vi "SubVI_Res_Result.vi"(8 "error in":errorcluster caption="에러 입력(에러 없음)", 11 "Q_data":T1) -> (0 "error out":errorcluster caption="에러 출력")   [LabVIEW 2016]
uses:
  Ctrls/raw Q data.ctl
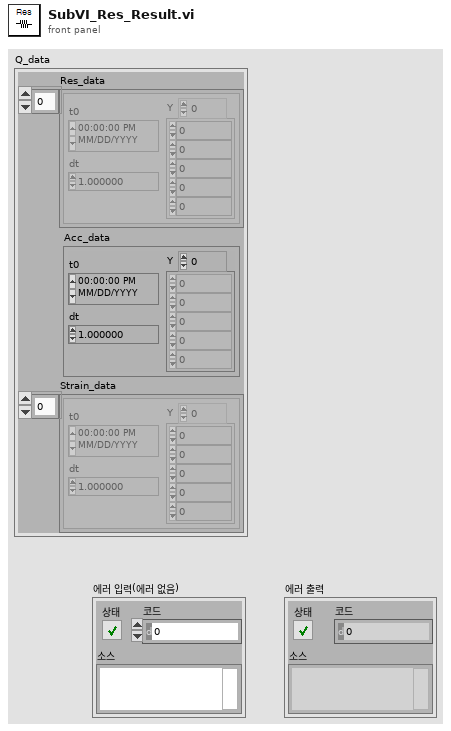
[diagram p1: front panel]
types:
  T1 = typedef "raw Q data.ctl" = cluster{"Res_data":waveform(dbl)[], "Acc_data":waveform(dbl), "Strain_data":waveform(dbl)[]}
  T2 = cluster{"[0]":dbl, "[1]":dbl, "[2]":dbl, "[3]":dbl, "[4]":dbl, "[5]":dbl, "[6]":dbl, "[7]":dbl, "[8]":dbl, "[9]":dbl, "[10]":dbl, "[11]":dbl, "[12]":dbl, "[13]":dbl, "[14]":dbl}
  T3 = cluster{"Num":u32[], "Resister 1~5":u8[][], "Resister 6~10":u8[][], "Resister 11~15":u8[][]}
  T4 = typedef "raw data type.ctl" = cluster{"Resistor values":cluster{"[0]":dbl, "[1]":dbl, "[2]":dbl, "[3]":dbl, "[4]":dbl, "[5]":dbl, "[6]":dbl, "[7]":dbl, "[8]":dbl, "[9]":dbl, "[10]":dbl, "[11]":dbl, "[12]":dbl, "[13]":dbl, "[14]":dbl}, "Resistor tables":u8[], "Pass Fails":bool[]}
  T5 = typedef "Total data.ctl" = cluster{"Raw Data":T1, "Resister result data":T4, "Result Table update":cluster{"Num":u32[], "Resister 1~5":u8[][], "Resister 6~10":u8[][], "Resister 11~15":u8[][]}, "Strain Data":cluster{"Strain 1":dbl, "Strain 2":dbl, "Strain 3":dbl, "Strain 4":dbl}, "Acc Result":cluster{"Acc Peak":dbl, "Acc time":dbl, "Acc area":dbl}, "STATUS":cluster{"status":string, "all_fail":bool, "emg":bool, "cycle":u16, "file name":string}, "Speed":dbl, "Acc peak time":dbl, "Max Strain":dbl, "Resistor at peak":cluster{"[0]":dbl, "[1]":dbl, "[2]":dbl, "[3]":dbl, "[4]":dbl, "[5]":dbl, "[6]":dbl, "[7]":dbl, "[8]":dbl, "[9]":dbl, "[10]":dbl, "[11]":dbl, "[12]":dbl, "[13]":dbl, "[14]":dbl}, "Acc peak index":u32, "time":string, "Cycle finish":bool, "Resistor at ini":cluster{"[0]":dbl, "[1]":dbl, "[2]":dbl, "[3]":dbl, "[4]":dbl, "[5]":dbl, "[6]":dbl, "[7]":dbl, "[8]":dbl, "[9]":dbl, "[10]":dbl, "[11]":dbl, "[12]":dbl, "[13]":dbl, "[14]":dbl}}
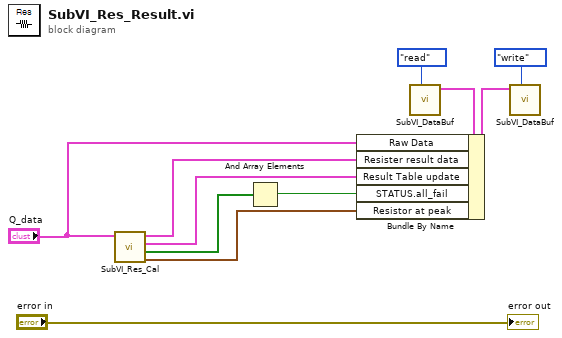
[diagram p0: block diagram]
diagram:
  n1 = call "SubVI_Res_Cal.vi"("Q_data"="Q_data") -> ("Max Resistor"=w2:T2, "PassFail"=w3:bool[], "Result Table update"=w4:T3, "Resister result data"=w7:T4)  [unwired: 7 in]
  n2 = And Array Elements(Boolean array=w3) -> (logical AND=w5:bool)
  n3 = call "SubVI_DataBuf.vi"("cmd"=enum16{"ini", "write", "read"}."read") -> ("Total data 2"=w6:T5)  [unwired: 9 in, 1 out]
  n4 = Bundle By Name(cluster=w6, "Raw Data"="Q_data", "Resister result data"=w7, "Result Table update"=w4, "STATUS.all_fail"=w5, "Resistor at peak"=w2) -> (w8:T5)
  n5 = call "SubVI_DataBuf.vi"("cmd"=enum16{"ini", "write", "read"}."write", "Total data"=w8) -> ()  [unwired: 8 in, 2 out]
  "error out" <- "error in"
